vi "Build.vi"(0 "Compound_Installer In":refnum<class "Compound_Installer.lvclass">) -> (4 "Compound_Installer Out":refnum<class "Compound_Installer.lvclass">)   [LabVIEW 2017, in "CL_G3_VIComponentBuilder.lvlib" / "Compound_Installer.lvclass"]
doc: "Creates the export artifacts, such as an executable, VI Package, DLL, etc."
uses:
  Compound_Installer.lvclass
  C:/Tool Chain Support/Software Module Builder/Source/Exports/Exports/Export.lvclass
  Exports/Export.lvclass/Export.ctl
  Compound_Installer.lvclass/Compound_Installer.ctl
  Exports/Accessors/Read Export Operation Errors.vi
  Exports/Accessors/Write Export Operation Errors.vi
  Accessors/Read Sub Export Build Order.vi
  Exports/Export.lvclass
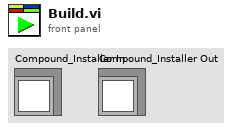
[diagram p1: front panel]
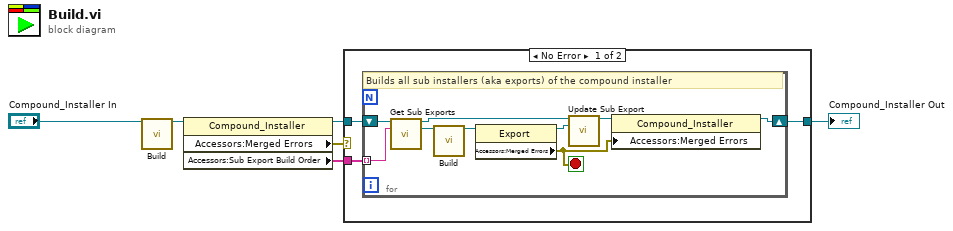
[diagram p0: block diagram]
diagram:
  n1 = call-parent "Build.vi"("Export In"="Compound_Installer In") -> ("Export Out"=w2:refnum<class "Compound_Installer.lvclass">)  [unwired: 14 in]
  n2 = property class="Compound_Installer"(reference=w2) -> (reference out=w4:refnum<class "Compound_Installer.lvclass">, "Accessors:Merged Errors"=w1:errorcluster, "Accessors:Sub Export Build Order"=w3:string[])  [unwired: 1 in, 1 out]
  n3 = case shown="No Error" w1 {
    tunnel: [w9 w19] -> w5
    tunnel: w4 -> [w8 w19]
    tunnel: w3 -> [w7 _]
    frame No Error {
      n4 = for {
        shift-right: [w11] -> w9
        shift-left: w8 -> [w18]
        tunnel: w7 -> [w16] mode=indexing
        stop <- w10 stop-if-true
        # "Builds all sub installers (aka exports) of the compound installer"
        n5 = call-dynamic "Get Sub Exports.vi"("NSIS_Installer in"=w18, "Sub Installer Name"=w16) -> ("NSIS_Installer out"=w15:refnum<class "Compound_Installer.lvclass">, "Export"=w17:refnum<class "Export.lvclass">)  [unwired: 10 in, 2 out]
        n6 = call-dynamic "Build.vi"("Export In"=w17) -> ("Export Out"=w13:refnum<class "Export.lvclass">)  [unwired: 14 in]
        n7 = property class="Export"(reference=w13) -> (reference out=w12:refnum<class "Export.lvclass">, "Accessors:Merged Errors"=w10:errorcluster)  [unwired: 1 in, 1 out]
        n8 = call-dynamic "Update Sub Export.vi"("NSIS_Installer in"=w15, "Sub Export"=w12) -> ("NSIS_Installer out"=w14:refnum<class "Compound_Installer.lvclass">)  [unwired: 12 in, 1 out]
        n9 = property class="Compound_Installer"(reference=w14, "Accessors:Merged Errors"=w10) -> (reference out=w11:refnum<class "Compound_Installer.lvclass">)  [unwired: 1 in, 1 out]
      }
    }
    frame Error {
    }
  }
  "Compound_Installer Out" <- w5
